vi "Error log.vi"(11 "Error in":errorcluster) -> (0 "Error Log Table":string[][](table), 15 "Error out":errorcluster)   [LabVIEW 2020, in "PSRR Monitor.lvlib"]
doc: "This VI is used to get the error log of the PSRR monitor and the error wiill be visualize only of the error log is enabled"
uses:
  PSRR Monitor.lvlib
  Typedefs/User LV2 operations.ctl
  <vilib>/Utility/miscctls.llb/LVRowAndColumnUnsignedTypeDef.ctl
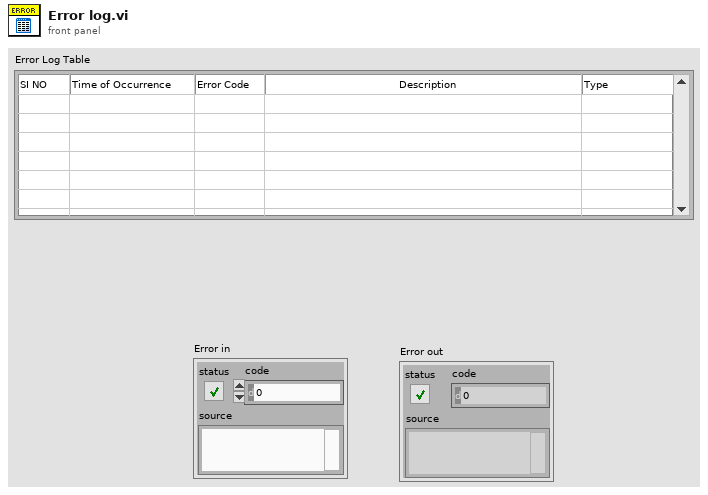
[diagram p1: front panel]
types:
  T1 = typedef "PSRR Monitor.lvlib/User LV2 operations.ctl" = enum16{"Destroy", "Get ref", "Generate", "Create"}
  T2 = typedef "LVRowAndColumnUnsignedTypeDef.ctl" = cluster{"Row":u32, "Column":u32}
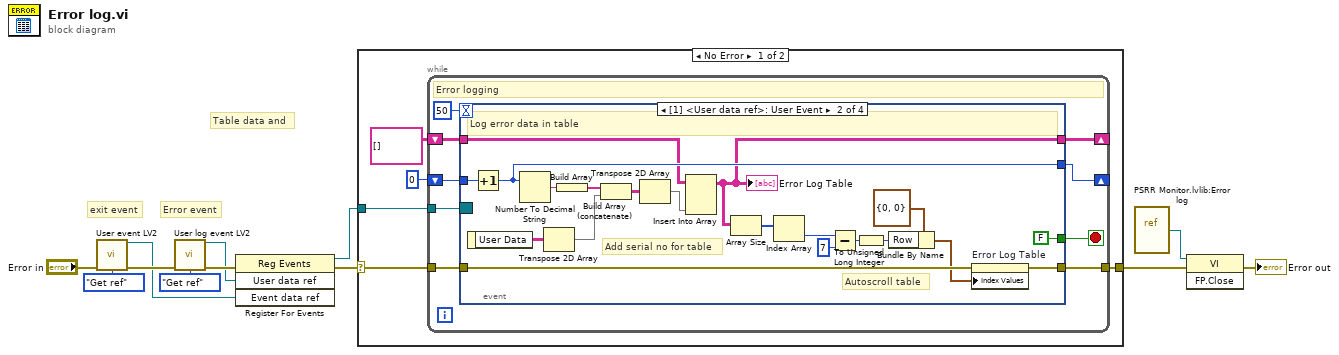
[diagram p0: block diagram]
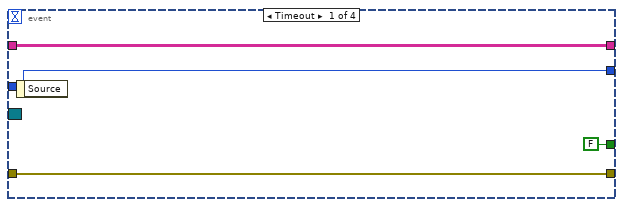
[diagram p2: hidden frame]
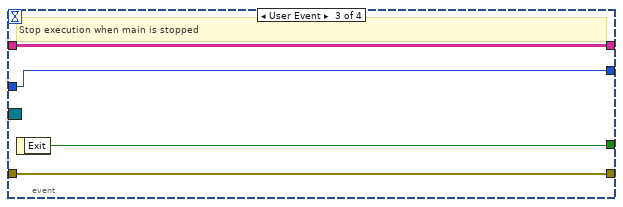
[diagram p3: hidden frame]
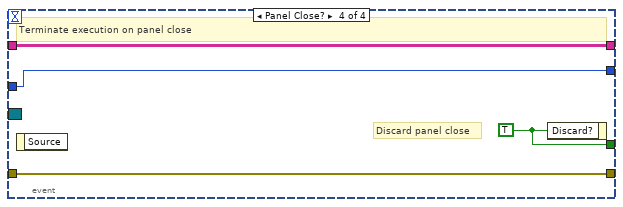
[diagram p4: hidden frame]
diagram:
  # "Table data and"
  # "exit event"
  # "Error event"
  n1 = call "User event LV2.vi"("Error in"="Error in", "Operation"=User_LV2_operations."Get ref") -> ("Event data ref"=w5:refnum<user-event>, "Error out"=w10:errorcluster)  [unwired: 12 in]
  n2 = call "User log event LV2.vi"("Error in"=w10, "Operation"=User_LV2_operations."Get ref") -> ("User data ref"=w6:refnum<user-event>, "Error out"=w8:errorcluster)  [unwired: 12 in]
  n3 = register-events(error in=w8, w6, w5) -> (reference out=w4:refnum<event-registration>, error out=w7:errorcluster)  [unwired: 1 in]
  n4 = case shown="No Error" w7 {
    selector: w7 -> [w17 w59]
    tunnel: [w16 w59] -> w2
    tunnel: w4 -> [w15 _]
    frame No Error {
      n5 = while {
        tunnel: w17 -> [w25]
        tunnel: [w26] -> w16
        tunnel: w15 -> [w23]
        shift-right: [w21] -> _
        shift-left: 0 -> [w22]
        shift-right: [w19] -> _
        shift-left: string[][] [] ("transposed array") -> [w20]
        stop <- w24 stop-if-true
        # "Error logging"
        n6 = event shown="[1] <User data ref>: User Event" {
          selector: w23 -> [_ _ _ _]
          dyn-events: _ -> [_ _ _ _]
          timeout: 50 -> [_ _ _ _]
          tunnel: [w30 w39 w53 w57] -> w26
          tunnel: w25 -> [w30 w40 w53 w57]
          tunnel: [FALSE ("Discard?") FALSE ("Discard?") w54 w58] -> w24
          tunnel: w22 -> [w28 w49 w52 w56]
          tunnel: [w28 w48 w52 w56] -> w21
          tunnel: w20 -> [w27 w42 w51 w55]
          tunnel: [w27 w38 w51 w55] -> w19
          event Timeout {
            n7 = event-data() -> ()  [unwired: 1 in, 1 out]
          }
          event User Event {
            # "Autoscroll table"
            # "Add serial no for table"
            # "Log error data in table"
            n8 = event-data() -> ("User Data"=w45:string[][])  [unwired: 1 in]
            n9 = Increment(x=w49) -> (x+1=w48:i32)
            n10 = Number To Decimal String(number=w48) -> (decimal integer string=w47:string)  [unwired: 1 in]
            n11 = Transpose 2D Array(2D array=w45) -> (transposed array=w44:string[][])
            n12 = Build Array(w47) -> (w46:string[])
            n13 = Build Array (concatenate)(w46, w44) -> (w43:string[][])
            n14 = Transpose 2D Array(2D array=w43) -> (transposed array=w41:string[][])
            n15 = Insert Into Array(array=w42, new element=w41) -> (w38:string[][])  [unwired: 2 in]
            "Error Log Table" <- w38
            n16 = Array Size(array=w38) -> (size(s)=w37:i32[])
            n17 = Index Array(array=w37) -> (element=w35:i32)  [unwired: 1 in]
            n18 = Subtract(x=w35, y=7) -> (x-y=w32:i32)
            n19 = To Unsigned Long Integer(number=w32) -> (unsigned 32bit integer=w33:u32)
            n20 = Bundle By Name(cluster=T2 {"Row"=0, "Column"=0} ("Index Values"), "Row"=w33) -> (w31:T2)
            n21 = property on="Error Log Table" class="Tbl (strict)"(error in=w40, "Index Values"=w31) -> (error out=w39:errorcluster)  [unwired: 1 in, 1 out]
          }
          event User Event {
            # "Stop execution when main is stopped"
            n22 = event-data() -> ("Exit"=w54:bool)  [unwired: 1 in]
          }
          event Panel Close? {
            w58 = TRUE ("Discard?")
            # "Discard panel close"
            # "Terminate execution on panel close"
            n23 = event-data() -> ()  [unwired: 1 in, 1 out]
            n24 = event-data("Discard?"=w58) -> ()  [unwired: 1 in, 1 out]
          }
        }
      }
    }
    frame Error {
    }
  }
  n25 = vi-ref "PSRR Monitor.lvlib:Error log.vi"() -> (w3:refnum<vi>)
  n26 = invoke class="VI" method="FP.Close"(reference=w3, error in=w2) -> (error out=→"Error out":errorcluster)  [unwired: 1 in, 2 out]
